vi "Serial Daemon.vi"(8 "UUID":string, 9 "data model":refnum<class "Device Data Model.lvclass">, 10 "transmission data unit":refnum<class "Transmission Data Unit.lvclass">, 11 "serial slave":refnum<class "Serial Slave.lvclass">) -> ()   [LabVIEW 2017, in "SubVIs.lvlib" / "Serial Slave.lvclass"]
uses:
  <vilib>/Modbus/subvis/Protocol/Serial/Serial Slave/Serial Slave.lvclass
  <vilib>/Modbus/subvis/Transmission Data Unit (ADU)/Transmission Data Unit/Transmission Data Unit.lvclass
  C:/builds/penguin/iak/lvdsc/trunk/17.0/lv/vi.lib/Modbus/subvis/Protocol/Interfaces/Network Slave/Network Slave.lvclass
  C:/builds/penguin/iak/lvdsc/trunk/17.0/lv/vi.lib/Modbus/subvis/Protocol/Interfaces/Network Protocol/Network Protocol.lvclass
  <vilib>/Modbus/subvis/Data and Functions/Device Data Model/Device Data Model.lvclass
  <vilib>/Modbus/subvis/Protocol/Interfaces/Network Slave/Network Slave.lvclass/Network Slave.ctl
  <vilib>/Modbus/subvis/Protocol/Serial/Serial Slave/Serial Slave.lvclass/Serial Slave.ctl
  <vilib>/Modbus/subvis/Protocol/Interfaces/Network Slave/Network Slave.lvclass
panel:
  in  "stop":bool
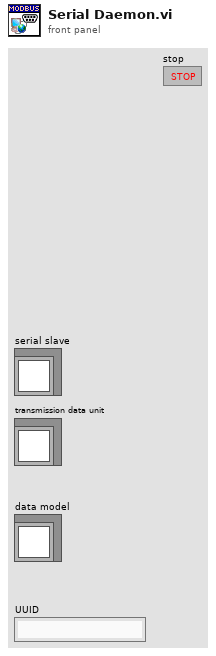
[diagram p1: front panel]
types:
  T1 = enum16{"Not Started", "Running", "Error", "Stopped"}
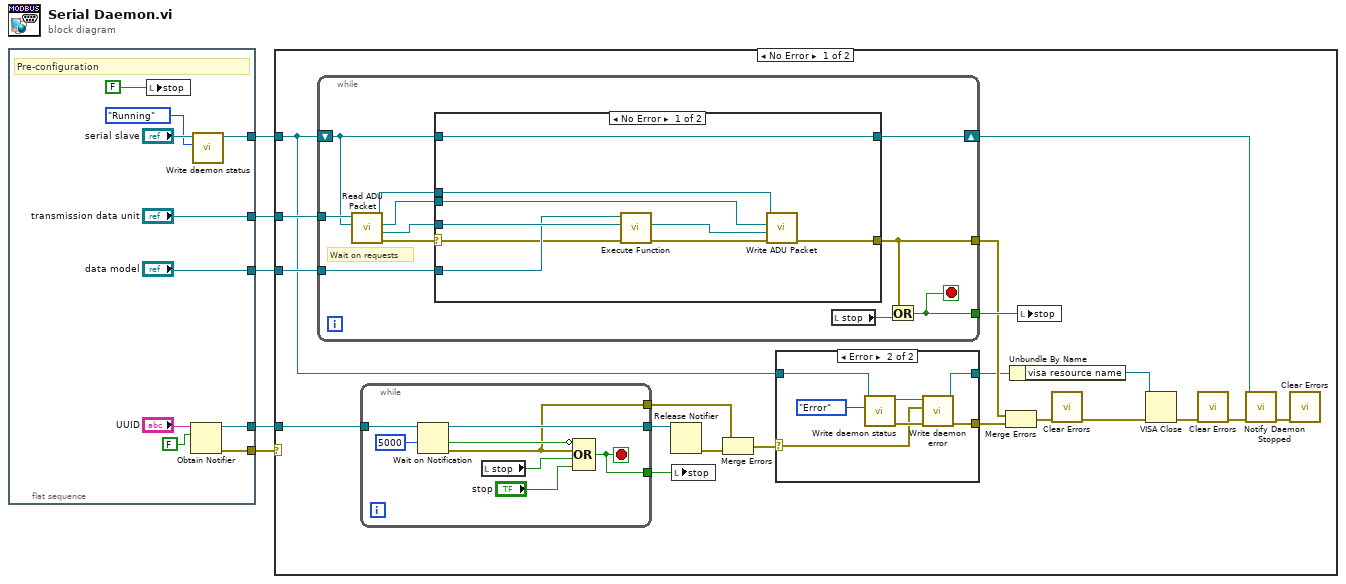
[diagram p0: block diagram]
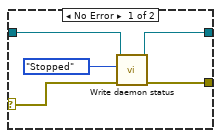
[diagram p2: hidden frame]
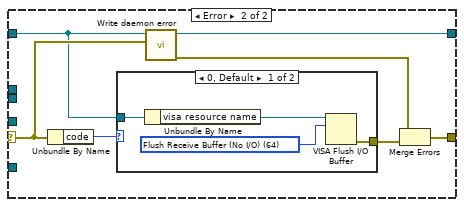
[diagram p3: hidden frame]
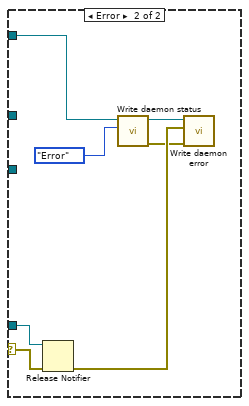
[diagram p5: hidden frame]
diagram:
  n1 = flat-sequence {
    tunnel: [w8] -> w1
    tunnel: ["transmission data unit"] -> w5
    tunnel: ["data model"] -> w4
    tunnel: [w14] -> w3
    tunnel: [w13] -> w2
    frame #0 {
      # "Pre-configuration"
      n2 = local write "stop"(FALSE ("stop")) -> ()
      n3 = Obtain Notifier(name (unnamed)="UUID", notification data type=FALSE) -> (notifier out=w13:refnum<notifier>, error out=w14:errorcluster)  [unwired: 2 in, 1 out]
      n4 = call <vilib>:"Write daemon status.vi"("daemon status"=T1."Running", "network slave in"="serial slave") -> ("network slave out"=w8:refnum<class "Serial Slave.lvclass">)  [unwired: 8 in, 1 out]
    }
  }
  n5 = case shown="No Error" w3 {
    selector: w3 -> [_ w93]
    tunnel: w5 -> [w35 _]
    tunnel: w4 -> [w34 _]
    tunnel: w1 -> [w29 w91]
    tunnel: w2 -> [w32 w92]
    frame No Error {
      n6 = while {
        tunnel: w35 -> [w66]
        tunnel: w34 -> [w64]
        tunnel: [w61] -> w33
        tunnel: [w57] -> w28
        shift-right: [w56] -> w19
        shift-left: w29 -> [w58]
        stop <- w61 stop-if-true
        # "Wait on requests"
        n7 = call-dynamic "Read ADU Packet.vi"("protocol layer"=w58, "transmission data unit in"=w66) -> ("error out"=w65:errorcluster, "Modbus data unit"=w60:refnum<class "Modbus Data Unit (PDU).lvclass">, "protocol layer out"=w59:refnum<class "Network Protocol.lvclass">, "transmission data unit out"=w63:refnum<class "Transmission Data Unit.lvclass">)  [unwired: 5 in, 1 out]
        n8 = case shown="No Error" w65 {
          selector: w65 -> [w69 w81]
          tunnel: w64 -> [w70 _]
          tunnel: w63 -> [w75 _]
          tunnel: w60 -> [w74 _]
          tunnel: w59 -> [w71 _]
          tunnel: w58 -> [w67 w80]
          tunnel: [w68 w77] -> w57
          tunnel: [w67 w76] -> w56
          frame No Error {
            n9 = call-dynamic "Execute Function.vi"("error in (no error)"=w69, "Modbus request"=w74, "device data model in"=w70) -> ("error out"=w72:errorcluster, "Modbus response"=w73:refnum<class "Modbus Data Unit (PDU).lvclass">)  [unwired: 6 in, 1 out]
            n10 = call-dynamic "Write ADU Packet.vi"("error in (no error)"=w72, "Modbus data unit"=w73, "protocol layer"=w71, "transmission data unit in"=w75) -> ("error out"=w68:errorcluster)  [unwired: 5 in, 2 out]
          }
          frame Error {
            n11 = Unbundle By Name(w81) -> ("code"=w82:i32)
            n12 = case shown="0, Default" w82 {
              tunnel: w80 -> [w86 _]
              tunnel: [w83 _] -> w79
              frame 0, Default {
                w84 = u16 64 items=["Flush Receive Buffer"=16, "Write Transmit Buffer to Device"=32, "Flush Receive Buffer (No I/O)"=64, "Flush Transmit Buffer"=128] ("Mask")
                n13 = Unbundle By Name(w86) -> ("visa resource name"=w85:refnum<visa-resource-name>)
                n14 = VISA Flush I/O Buffer(VISA resource name=w85, mask (16)=w84) -> (error out=w83:errorcluster)  [unwired: 1 in, 1 out]
              }
              frame 56 {
              }
            }
            n15 = call <vilib>:"Write daemon error.vi"("daemon error"=w81, "network slave in"=w80) -> ("error out"=w78:errorcluster, "network slave out"=w76:refnum<class "Serial Slave.lvclass">)  [unwired: 8 in]
            n16 = Merge Errors(w78, w79) -> (w77:errorcluster)
          }
        }
        n17 = local read "stop"() -> (w62:bool)
        n18 = Or(x=w57, y=w62) -> (x .or. y?=w61:bool)
      }
      n19 = while {
        tunnel: w32 -> [w54]
        tunnel: [w53] -> w30
        tunnel: [w49] -> w31
        tunnel: [w48] -> w21
        stop <- w49 stop-if-true
        n20 = Wait on Notification(notifier=w54, timeout in ms (-1)=5000) -> (notifier out=w53:refnum<notifier>, timed out?=w52:bool, error out=w48:errorcluster)  [unwired: 2 in, 1 out]
        n21 = local read "stop"() -> (w51:bool)
        n22 = Compound Arithmetic op=OR(invert w52, w48, w51, "stop") -> (w49:bool)
      }
      n23 = Release Notifier(notifier=w30) -> (error out=w20:errorcluster)  [unwired: 2 in, 2 out]
      n24 = local write "stop"(w31) -> ()
      n25 = Merge Errors(w21, w20) -> (w22:errorcluster)
      n26 = case shown="Error" w22 {
        selector: w22 -> [w39 w43]
        tunnel: w29 -> [w38 w45]
        tunnel: [w37 w42] -> w27
        tunnel: [w36 w41] -> w25
        frame No Error {
          n27 = call <vilib>:"Write daemon status.vi"("error in (no error)"=w39, "daemon status"=T1."Stopped", "network slave in"=w38) -> ("error out"=w37:errorcluster, "network slave out"=w36:refnum<class "Serial Slave.lvclass">)  [unwired: 7 in]
        }
        frame Error {
          n28 = call <vilib>:"Write daemon status.vi"("daemon status"=T1."Error", "network slave in"=w45) -> ("error out"=w46:errorcluster, "network slave out"=w47:refnum<class "Serial Slave.lvclass">)  [unwired: 8 in]
          n29 = call <vilib>:"Write daemon error.vi"("error in (no error)"=w46, "daemon error"=w43, "network slave in"=w47) -> ("error out"=w42:errorcluster, "network slave out"=w41:refnum<class "Serial Slave.lvclass">)  [unwired: 7 in]
        }
      }
      n30 = Merge Errors(w28, w27) -> (w26:errorcluster)
      n31 = Unbundle By Name(w25) -> ("visa resource name"=w24:refnum<visa-resource-name>)
      n32 = local write "stop"(w33) -> ()
      n33 = call <vilib>:"Clear Errors.vi"("error in (no error)"=w26) -> ("error out"=w23:errorcluster)  [unwired: 5 in, 1 out]
      n34 = VISA Close(VISA resource name=w24, error in (no error)=w23) -> (error out=w17:errorcluster)
      n35 = call <vilib>:"Clear Errors.vi"("error in (no error)"=w17) -> ("error out"=w18:errorcluster)  [unwired: 5 in, 1 out]
      n36 = call <vilib>:"Notify Daemon Stopped.vi"("error in (no error)"=w18, "Network Slave in"=w19) -> ("error out"=w16:errorcluster)  [unwired: 8 in, 1 out]
      n37 = call <vilib>:"Clear Errors.vi"("error in (no error)"=w16) -> ()  [unwired: 5 in, 2 out]
    }
    frame Error {
      n38 = Release Notifier(notifier=w92, error in (no error)=w93) -> (error out=w88:errorcluster)  [unwired: 1 in, 2 out]
      n39 = call <vilib>:"Write daemon status.vi"("daemon status"=T1."Error", "network slave in"=w91) -> ("error out"=w87:errorcluster, "network slave out"=w89:refnum<class "Serial Slave.lvclass">)  [unwired: 8 in]
      n40 = call <vilib>:"Write daemon error.vi"("error in (no error)"=w87, "daemon error"=w88, "network slave in"=w89) -> ()  [unwired: 7 in, 2 out]
    }
  }
